vi "SECoP-unregisterUserError.vi"(8 "error in (no error)":errorcluster, 10 "registered SECoP error":T1 items=["warn: missing properties"=4, "warn: buffer too small"=3, "warn: custom property"=2, "warn: no description"=1, "success"=0, "error: unknown command"=-1, "error: invalid name"=-2, "error: invalid node"=-3, "error: invalid module"=-4, "error: invalid parameter"=-5, "error: invalid property"=-6, "error: invalid command"=-7, "error: not implemented"=-8, "error: readonly"=-9, "error: no data"=-10, "error: no memory"=-11, "error: not initialized"=-12, "error: invalid value"=-13, "error: missing mandatory prop"=-14, "error: no setter/getter"=-15, "error: no setter"=-16, "error: no getter"=-17, "error: name already in use"=-18], 11 "DLL path (in)":T2) -> (0 "error out":errorcluster, 3 "DLL path (out)":T2)   [LabVIEW 2023, in "SECoP.lvlib"]
doc: "Call <b>\"SECoP-unregisterUserError.vi\"</b> to undo the registration of \"SECoP-registerUserError.vi\".\n\n<b>DLL path</b> input and output of cluster from \"SECoP-Initialize.vi\"\n<b>registered SECoP error</b> previously registered \"SECoP-error.ctl\" code"
uses:
  SECoP.lvlib
  SECoP-libraries.ctl
  SECoP-error.ctl
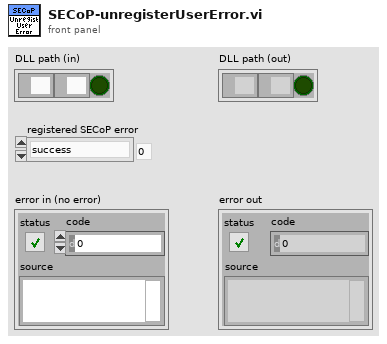
[diagram p1: front panel]
types:
  T1 = typedef "SECoP.lvlib/SECoP-error.ctl" = i32
  T2 = typedef "SECoP.lvlib/SECoP-libraries.ctl" = cluster{"serverDLL":path, "variantDLL":path, "cleanup_mode":bool}
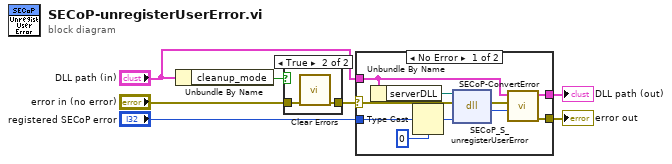
[diagram p0: block diagram]
diagram:
  n1 = Unbundle By Name("DLL path (in)") -> ("cleanup_mode"=w4:bool)
  n2 = case shown="True" w4 {
    tunnel: "error in (no error)" -> [w8 w10]
    tunnel: [w8 w9] -> w3
    frame False {
    }
    frame True {
      n3 = call <vilib>:"Clear Errors.vi"("error in (no error)"=w10) -> ("error out"=w9:errorcluster)  [unwired: 5 in, 1 out]
    }
  }
  n4 = case shown="No Error" w3 {
    selector: w3 -> [w19 w21]
    tunnel: "DLL path (in)" -> [w18 w22]
    tunnel: [w17 w22] -> w6
    tunnel: [w15 w21] -> w7
    tunnel: "registered SECoP error" -> [w13 _]
    frame No Error {
      n5 = Unbundle By Name(w18) -> ("serverDLL"=w20:path)
      n6 = Type Cast(type=0 ("iError"), x=w13) -> (*(type *) &x=w11:i32)
      n7 = dll-call lib="?" fn="SECoP_S_unregisterUserError"(path in=w20, error in=w19, "iError"=w11) -> (error out=w16:errorcluster, "return type"=w14:i32)  [unwired: 2 in, 1 out]
      n8 = call "SECoP-ConvertError.vi"("return code"=w14, "error in (no error)"=w16, "DLL path (in)"=w18) -> ("error out"=w15:errorcluster, "DLL path (out)"=w17:T2)  [unwired: 7 in]
    }
    frame Error {
    }
  }
  "DLL path (out)" <- w6
  "error out" <- w7
